vi "Send Cyclic to Main.vi"(8 "error in (no error)":errorcluster, 11 "CIFTemplatePlugin in":refnum<class "TemplatePlugin.lvclass">) -> (0 "error out":errorcluster, 3 "CIFTemplatePlugin out":refnum<class "TemplatePlugin.lvclass">)   [LabVIEW 2021, in "TemplatePlugin.lvclass"]
uses:
  TemplatePlugin.lvclass
  TemplatePlugin.lvclass/TemplatePlugin.ctl
  a548145f-fa5b-40dd-b142-8dd091c04010.vi
  <vilib>/CIF Foundation/CIF CIPC/SubVIs/Check Error.vi
  <vilib>/CIF Foundation/CIF CIPC/SubVIs/Get Element Write Position.vi
  <vilib>/CIF Foundation/CIF CIPC/SubVIs/Notify Of New Write.vi
  <vilib>/CIF Foundation/CIF CIPC/SubVIs/Get dll Path.vi
  <vilib>/CIF Foundation/CIF CIPC/SubVIs/Get Element Info Variant.vi
  <vilib>/Utility/error.llb/Trim Whitespace.vi
  <vilib>/Utility/error.llb/Error Cluster From Error Code.vi
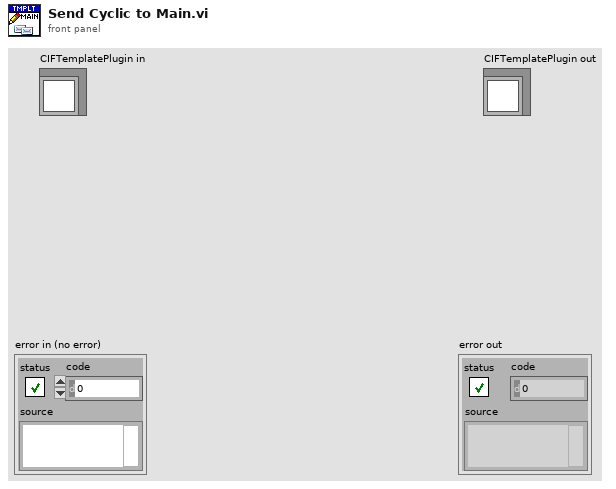
[diagram p1: front panel]
types:
  T1 = typedef "TemplateCommon.lvlib/To Main Cyclic Data.ctl" = cluster{"Data 1 -> Main":i32}
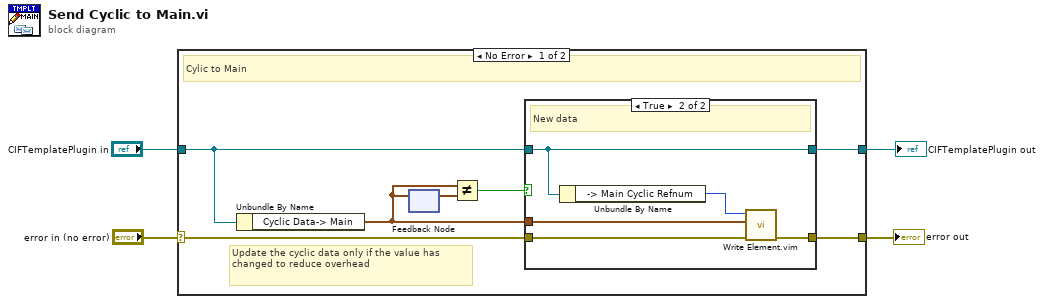
[diagram p0: block diagram]
diagram:
  n1 = case shown="No Error" "error in (no error)" {
    selector: "error in (no error)" -> [w5 w20]
    tunnel: [w8 w20] -> w3
    tunnel: [w9 w19] -> w1
    tunnel: "CIFTemplatePlugin in" -> [w7 w19]
    frame No Error {
      # "Update the cyclic data only if the value has changed to reduce overhead"
      # "Cylic to Main"
      n2 = Unbundle By Name(w7) -> ("Cyclic Data-> Main"=w10:T1)
      n3 = feedback-in #1(w10) -> ()
      n4 = feedback #1() -> (w11:T1)  [unwired: 1 in]
      n5 = Not Equal?(x=w10, y=w11) -> (x != y?=w6:bool)
      n6 = case shown="True" w6 {
        tunnel: w7 -> [w13 w18]
        tunnel: w10 -> [_ w16]
        tunnel: [w13 w18] -> w9
        tunnel: [w12 w14] -> w8
        tunnel: w5 -> [w12 w15]
        frame False {
        }
        frame True {
          # "New data"
          n7 = Unbundle By Name(w18) -> ("-> Main Cyclic Refnum"=w17:u64)
          n8 = call "Write Element.vim"("error in (no error)"=w15, "Data in"=w16, "CIPC Reference in"=w17) -> ("error out"=w14:errorcluster)  [unwired: 5 in, 3 out]
        }
      }
    }
    frame Error {
    }
  }
  "error out" <- w3
  "CIFTemplatePlugin out" <- w1
